vi "Localization.vi"(11 "Unlocalized":string) -> (3 "Localized":string)   [LabVIEW 2018, in "MWWL Verification Launcher.lvlib"]
doc: "This VI is used to provide localization -- that is, support for other human languages -- in the user interface. Given an input string, this VI returns the string that should be displayed for the current language. The idea is that you as a developer can use the Export/Import Strings feature of LabVIEW to produce a file that a translator can localize. The convention is that any control with \"DNL_\" as its label is skipped during localization (in English, this stands for Do Not Localize). The first array in this VI is one of these DNL_ controls. This array has the fixed strings that the program uses. The second array has the translated strings. Using this for all user visible text is sometimes cumbersome on the programmer, but it limits how many VIs have to be reviewed for localization.\n\nEven if you are not translating into other languages, this style of string lookup provides a central location for all your user visible text, which you may reuse at multiple points in your program, thus making it easy for tech writers to review for spelling or to make late-in-development-cycle changes with minimal risk to the rest of the code."
uses:
  MWWL Verification Launcher.lvlib
panel:
  in  "Localized Array":string[](array[string])=["MWWL Verification", "Loading Application...", "Reading Configuration File...", "Done!", "MWWL\r\nVerification", "Current Action:"]
  in  "DNL_Unlocalized Array":string[](array[string])=["Splash Screen Title", "Loading Application", "Reading Configuration", "Done!", "App Name", "Current Action:"]
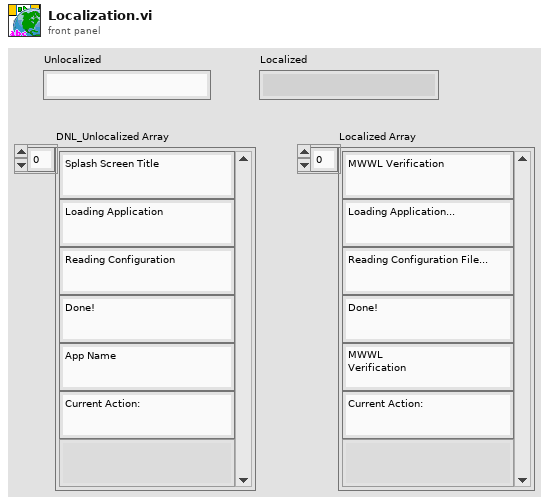
[diagram p1: front panel]
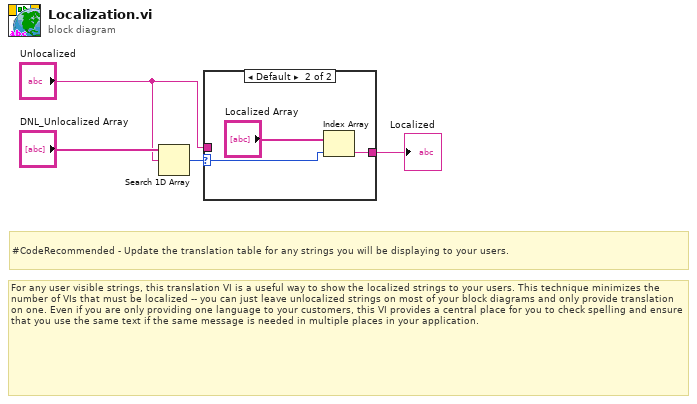
[diagram p0: block diagram]
diagram:
  # "#CodeRecommended - Update the translation table for any strings you will be displaying to your users."
  # "For any user visible strings, this translation VI is a useful way to show the localized strings to your users. This technique minimizes the number of VIs that must be localized -- you can just leave unlocalized strings on most of your block diagrams and only provide translation on one. Even if you are only providing one language to your customers, this VI provides a central place for you to check spelling and ensure that you use the same text if the same message is needed in multiple places in your application."
  n1 = Search 1D Array(1D array="DNL_Unlocalized Array", element="Unlocalized") -> (index of element=w2:i32)  [unwired: 1 in]
  n2 = case shown="Default" w2 {
    selector: w2 -> [_ w6]
    tunnel: [w5 w7] -> w3
    tunnel: "Unlocalized" -> [w5 _]
    frame ..-1 {
    }
    frame Default {
      n3 = Index Array(array="Localized Array", index=w6) -> (element=w7:string)
    }
  }
  "Localized" <- w3
